vi "Setup.vi"(8 "error in (no error)":errorcluster, 11 "UI View Test In":refnum<class "View Dev Test.lvclass">) -> (0 "error out":errorcluster, 3 "UI View Test Out":refnum<class "View Dev Test.lvclass">)   [LabVIEW 2020, in "View Dev Test.lvclass"]
uses:
  View Dev Test.lvclass
  C:/Git/astemes-triarc-framework/source/Framework Test/Base Class Test/Base Test.lvclass
  source/Framework/View/View.lvclass
  C:/Git/astemes-triarc-framework/source/Framework/Base/Base.lvclass
  source/Framework Test Suite/Base Class Test/Base Test.lvclass/Base Test.ctl
  View Dev Test.lvclass/View Dev Test.ctl
  source/Framework Test Suite/Base Class Test/Base Test.lvclass
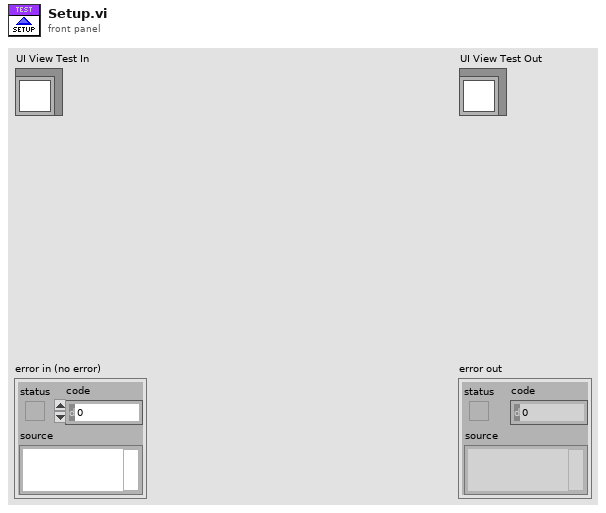
[diagram p1: front panel]
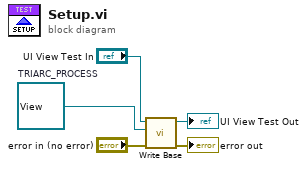
[diagram p0: block diagram]
diagram:
  w1 = refnum<class "View.lvclass"> refnum  # TRIARC_PROCESS
  n1 = call "Write Base.vi"("error in (no error)"="error in (no error)", "Base"=w1, "Base Class Test In"="UI View Test In") -> ("error out"=→"error out":errorcluster, "Base Class Test Out"=→"UI View Test Out":refnum<class "View Dev Test.lvclass">)  [unwired: 7 in]
